vi "Min Max Threads.vi"(8 "error in (no error)":errorcluster, 11 "lvzstd in":refnum<class "lvzstd.lvclass">) -> (0 "error out":errorcluster, 1 "max_count":i32, 2 "min_count":i32, 3 "lvzstd out":refnum<class "lvzstd.lvclass">)   [LabVIEW 2020, in "lvzstd.lvlib" / "lvzstd.lvclass"]
uses:
  lvzstd.lvclass
  lvzstd.lvclass/lvzstd.ctl
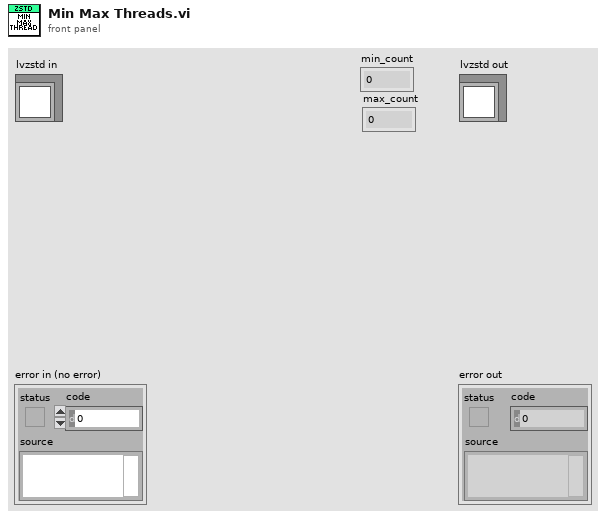
[diagram p1: front panel]
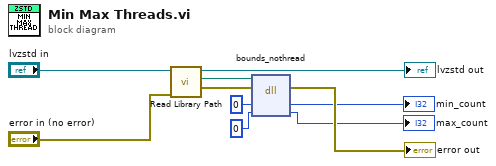
[diagram p0: block diagram]
diagram:
  n1 = call "Read Library Path.vi"("error in (no error)"="error in (no error)", "lvzstd in"="lvzstd in") -> ("error out"=w7:errorcluster, "Library Path"=w8:path, "lvzstd out"=→"lvzstd out":refnum<class "lvzstd.lvclass">)  [unwired: 7 in]
  n2 = dll-call lib="?" fn="bounds_nothread"(path in=w8, error in=w7, "min_count"=0, "max_count"=0 ("max_compressed_size")) -> (error out=→"error out":errorcluster, "min_count"=→"min_count":i32, "max_count"=→"max_count":i32)  [unwired: 2 in, 1 out]
